vi "KG set gas mfc.vi"(8 "Fehler (Eingang, kein Fehler)":errorcluster, 9 "gasname":string, 10 "mfc":u32, 11 "VISA-Ressourcenname":refnum<visa-resource-name>) -> (0 "Fehler (Ausgang)":errorcluster, 2 "Kommando gesendet":string, 3 "VISA-Ressourcenname (Ausgang)":refnum<visa-resource-name>)   [LabVIEW 2020, in "Linearisierung v2.lvlib" / "Gasteiler.lvlib" / "HovaCAL_Interface.lvlib" / "KGN.lvlib" / "set.lvlib"]
uses:
  set.lvlib
  KGN.lvlib
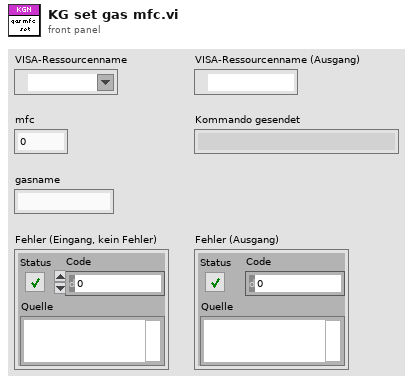
[diagram p1: front panel]
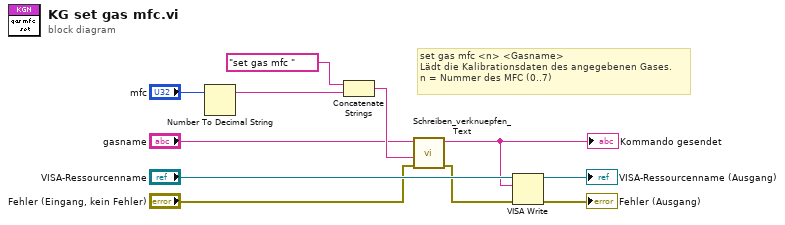
[diagram p0: block diagram]
diagram:
  # "set gas mfc <n> <Gasname>\nLädt die Kalibrationsdaten des angegebenen Gases.\nn = Nummer des MFC (0..7)"
  n1 = Number To Decimal String(number="mfc") -> (decimal integer string=w6:string)  [unwired: 1 in]
  n2 = Concatenate Strings("set gas mfc " ("Schreibpuffer"), w6) -> (w2:string)
  n3 = call "Schreiben_verknuepfen_Text.vi"("error in (no error)"="Fehler (Eingang, kein Fehler)", "Order"=w2, "parameter"="gasname") -> ("error out"=w4:errorcluster, "Verknüpfter String"=w3:string)  [unwired: 7 in]
  "Kommando gesendet" <- w3
  n4 = VISA Write(VISA resource name="VISA-Ressourcenname", write buffer=w3, error in (no error)=w4) -> (VISA resource name out=→"VISA-Ressourcenname (Ausgang)":refnum<visa-resource-name>, error out=→"Fehler (Ausgang)":errorcluster)  [unwired: 1 out]
